vi "CongaLine.vi"(0 "Type":T2, 11 "Mode":T1(ring)=enum."Static") -> (4 "vi reference":refnum<vi>, 6 "CReference Ctl":refnum<vi>, 8 "implemented?":bool, 15 "datatype image":picture)   [LabVIEW 2012, in "CRef.lvlib"]
uses:
  CRef.lvlib
  Core/Master Types.ctl
  Interface/CRef Numeric.llb/CRef Create Single.vi
  Interface/CRef Numeric.llb/CRef Get Single.vi
  Interface/CRef Numeric.llb/CRef Set Single.vi
  Interface/CRef Numeric.llb/CRef Static Single Reference.vi
  Interface/CRef Variant.llb/Variant CReference.ctl
  Interface/CRef Boolean.llb/Boolean CReference.ctl
  Interface/CRef Numeric.llb/U32 CReference.ctl
  Interface/CRef Numeric.llb/I32 CReference.ctl
  Interface/CRef Numeric.llb/Single CReference.ctl
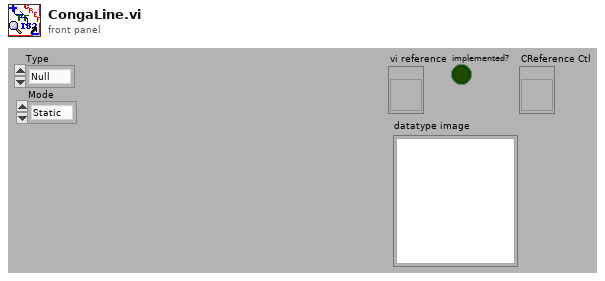
[diagram p1: front panel]
types:
  T1 = enum16{"Create", "Get", "Set", "Static", "Release"}
  T2 = typedef "CRef.lvlib/Master Types.ctl" = enum8{"Null", "Boolean", "U8", "I8", "U16", "I16", "U32", "I32", "U64", "I64", "Single", "Double", "Extended", "CSG", "CDB", "CXT", "Boolean(Def)", "U8(Def)", "I8(Def)", "U16(Def)", "I16(Def)", "U32(Def)", "I32(Def)", "Reserved Def", "Reserved Def1", "Single(Def)", "Double(Def)", "Reserved Def2", "Reserved Def3", "Reserved Def4", "Reserved Def5", "Unsigned(Def)", "Signed(Def)", "Real(Def)", "Reserved Def6", "Numeric(Def)", "String"}
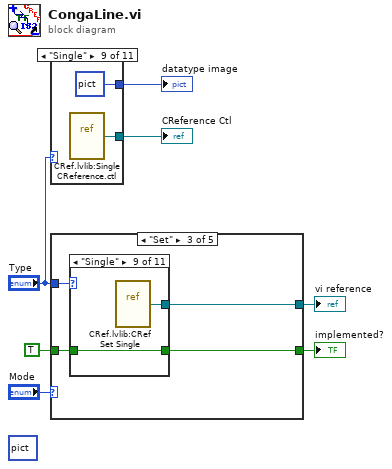
[diagram p0: block diagram]
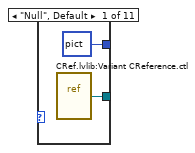
[diagram p2: hidden frame]
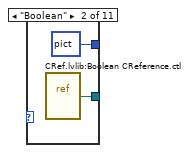
[diagram p3: hidden frame]
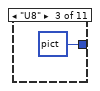
[diagram p4: hidden frame]
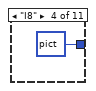
[diagram p5: hidden frame]
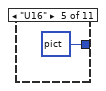
[diagram p6: hidden frame]
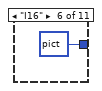
[diagram p7: hidden frame]
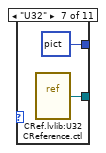
[diagram p8: hidden frame]
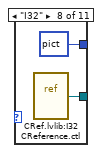
[diagram p9: hidden frame]
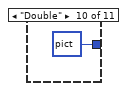
[diagram p10: hidden frame]
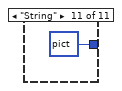
[diagram p11: hidden frame]
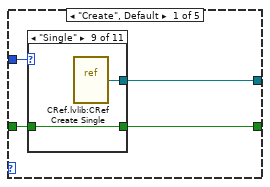
[diagram p12: hidden frame]
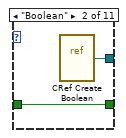
[diagram p14: hidden frame]
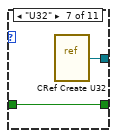
[diagram p19: hidden frame]
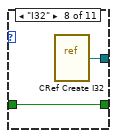
[diagram p20: hidden frame]
diagram:
  (unwired) picture bytes[534] ("new picture")
  n1 = case shown="\"Single\"" "Type" {
    tunnel: [picture bytes[558] ("new picture") picture bytes[534] ("new picture") picture bytes[534] ("new picture") picture bytes[534] ("new picture") picture bytes[534] ("new picture") picture bytes[534] ("new picture") picture bytes[534] ("new picture") picture bytes[534] ("new picture") picture bytes[534] ("new picture") picture bytes[534] ("new picture") picture bytes[534] ("new picture")] -> w3
    tunnel: [w8 w10 _ _ _ _ w16 w18 w20 _ _] -> w1
    frame "Null", Default {
      n2 = vi-ref "CRef.lvlib:Variant CReference.ctl"() -> (w8:refnum<vi>)
    }
    frame "Boolean" {
      n3 = vi-ref "CRef.lvlib:Boolean CReference.ctl"() -> (w10:refnum<vi>)
    }
    frame "U8" {
    }
    frame "I8" {
    }
    frame "U16" {
    }
    frame "I16" {
    }
    frame "U32" {
      n4 = vi-ref "CRef.lvlib:U32 CReference.ctl"() -> (w16:refnum<vi>)
    }
    frame "I32" {
      n5 = vi-ref "CRef.lvlib:I32 CReference.ctl"() -> (w18:refnum<vi>)
    }
    frame "Single" {
      n6 = vi-ref "CRef.lvlib:Single CReference.ctl"() -> (w20:refnum<vi>)
    }
    frame "Double" {
    }
    frame "String" {
    }
  }
  "datatype image" <- w3
  "CReference Ctl" <- w1
  n7 = case shown="\"Set\"" "Mode" {
    tunnel: "Type" -> [w27 w39 w51 w63 _]
    tunnel: [w26 w38 w50 w62 w73] -> w6
    tunnel: TRUE -> [w25 w37 w49 w61 w72]
    tunnel: [w24 w36 w48 w60 w72] -> w4
    frame "Create", Default {
      n8 = case shown="\"Single\"" w27 {
        tunnel: [_ w29 _ _ _ _ w31 w33 w35 _ _] -> w26
        tunnel: w25 -> [_ w28 _ _ _ _ w30 w32 w34 _ _]
        tunnel: [_ w28 _ _ _ _ w30 w32 w34 _ _] -> w24
        frame "Null", Default {
        }
        frame "Boolean" {
          n9 = vi-ref "CRef Create Boolean.vi"() -> (w29:refnum<vi>)
        }
        frame "U8" {
        }
        frame "I8" {
        }
        frame "U16" {
        }
        frame "I16" {
        }
        frame "U32" {
          n10 = vi-ref "CRef Create U32.vi"() -> (w31:refnum<vi>)
        }
        frame "I32" {
          n11 = vi-ref "CRef Create I32.vi"() -> (w33:refnum<vi>)
        }
        frame "Single" {
          n12 = vi-ref "CRef.lvlib:CRef Create Single.vi"() -> (w35:refnum<vi>)
        }
        frame "Double" {
        }
        frame "String" {
        }
      }
    }
    frame "Get" {
      n13 = case shown="\"Single\"" w39 {
        tunnel: [_ w41 _ _ _ _ w43 w45 w47 _ _] -> w38
        tunnel: w37 -> [_ w40 _ _ _ _ w42 w44 w46 _ _]
        tunnel: [_ w40 _ _ _ _ w42 w44 w46 _ _] -> w36
        frame "Null", Default {
        }
        frame "Boolean" {
          n14 = vi-ref "CRef Get Boolean.vi"() -> (w41:refnum<vi>)
        }
        frame "U8" {
        }
        frame "I8" {
        }
        frame "U16" {
        }
        frame "I16" {
        }
        frame "U32" {
          n15 = vi-ref "CRef Get U32.vi"() -> (w43:refnum<vi>)
        }
        frame "I32" {
          n16 = vi-ref "CRef Get I32.vi"() -> (w45:refnum<vi>)
        }
        frame "Single" {
          n17 = vi-ref "CRef.lvlib:CRef Get Single.vi"() -> (w47:refnum<vi>)
        }
        frame "Double" {
        }
        frame "String" {
        }
      }
    }
    frame "Set" {
      n18 = case shown="\"Single\"" w51 {
        tunnel: [_ w53 _ _ _ _ w55 w57 w59 _ _] -> w50
        tunnel: [_ w52 _ _ _ _ w54 w56 w58 _ _] -> w48
        tunnel: w49 -> [_ w52 _ _ _ _ w54 w56 w58 _ _]
        frame "Null", Default {
        }
        frame "Boolean" {
          n19 = vi-ref "CRef Set Boolean.vi"() -> (w53:refnum<vi>)
        }
        frame "U8" {
        }
        frame "I8" {
        }
        frame "U16" {
        }
        frame "I16" {
        }
        frame "U32" {
          n20 = vi-ref "CRef Set U32.vi"() -> (w55:refnum<vi>)
        }
        frame "I32" {
          n21 = vi-ref "CRef Set I32.vi"() -> (w57:refnum<vi>)
        }
        frame "Single" {
          n22 = vi-ref "CRef.lvlib:CRef Set Single.vi"() -> (w59:refnum<vi>)
        }
        frame "Double" {
        }
        frame "String" {
        }
      }
    }
    frame "Static" {
      n23 = case shown="\"Single\"" w63 {
        tunnel: [_ w65 _ _ _ _ w67 w69 w71 _ _] -> w62
        tunnel: [_ w64 _ _ _ _ w66 w68 w70 _ _] -> w60
        tunnel: w61 -> [_ w64 _ _ _ _ w66 w68 w70 _ _]
        frame "Null", Default {
        }
        frame "Boolean" {
          n24 = vi-ref "CRef Static Boolean Reference.vi"() -> (w65:refnum<vi>)
        }
        frame "U8" {
        }
        frame "I8" {
        }
        frame "U16" {
        }
        frame "I16" {
        }
        frame "U32" {
          n25 = vi-ref "CRef Static U32 Reference.vi"() -> (w67:refnum<vi>)
        }
        frame "I32" {
          n26 = vi-ref "CRef Static I32 Reference.vi"() -> (w69:refnum<vi>)
        }
        frame "Single" {
          n27 = vi-ref "CRef.lvlib:CRef Static Single Reference.vi"() -> (w71:refnum<vi>)
        }
        frame "Double" {
        }
        frame "String" {
        }
      }
    }
    frame "Release" {
      n28 = vi-ref "CRef Release Address.vi"() -> (w73:refnum<vi>)
    }
  }
  "vi reference" <- w6
  "implemented?" <- w4
